vi "Save.vi"(11 "Cerebellum in":refnum<class "Cerebellum.lvclass">) -> (0 "error out":errorcluster, 3 "File name":string)   [LabVIEW 2016, in "Cerebellum.lvclass"]
uses:
  Cerebellum.lvclass
  <vilib>/Utility/xml.llb/Write to XML File(string).vi
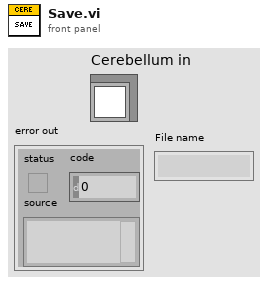
[diagram p1: front panel]
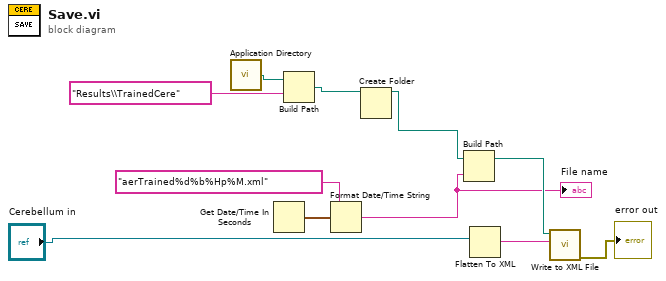
[diagram p0: block diagram]
diagram:
  n1 = call <vilib>:"Application Directory.vi"() -> ("Application Directory"=w5:path)
  n2 = Get Date/Time In Seconds() -> (seconds since 1Jan1904=w11:timestamp)
  n3 = Build Path(base path=w5, name or relative path="Results\\TrainedCere") -> (appended path=w4:path)
  n4 = Format Date/Time String(time format string (%c)="aerTrained%d%b%Hp%M.xml", seconds (now)=w11) -> (date/time string=w7:string)  [unwired: 1 in]
  "File name" <- w7
  n5 = Create Folder(path (use dialog)=w4) -> (created path=w3:path)  [unwired: 2 in, 2 out]
  n6 = Build Path(base path=w3, name or relative path=w7) -> (appended path=w8:path)
  n7 = Flatten To XML(anything="Cerebellum in") -> (xml string=w9:string)
  n8 = call-poly <vilib>:"Write to XML File.vi"("XML Input"=w9, "XML File Path"=w8) -> ("error out"=→"error out":errorcluster)  [unwired: 7 in, 2 out]
